vi "Release.vi"(8 "error in (no error)":errorcluster, 11 "Sequence in":refnum<class "Sequence.lvclass">) -> (0 "error out":errorcluster)   [LabVIEW 2020, in "TSnax.lvlib" / "Sequence.lvclass"]
uses:
  Sequence.lvclass
  Sequence.lvclass/Sequence.ctl
  PropertyObject/PropertyObject.lvclass
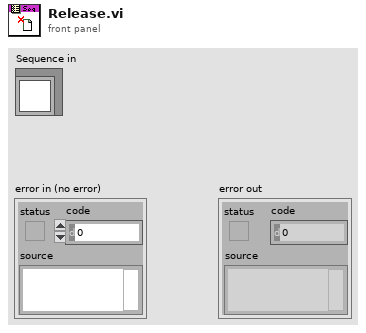
[diagram p1: front panel]
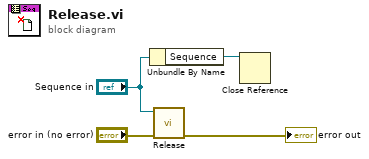
[diagram p0: block diagram]
diagram:
  n1 = Unbundle By Name("Sequence in") -> ("Sequence"=w1:refnum<k7>)
  n2 = call-parent "Release.vi"("error in (no error)"="error in (no error)", "PropertyObject in"="Sequence in") -> ("error out"=→"error out":errorcluster)  [unwired: 9 in]
  n3 = Close Reference(reference=w1) -> ()  [unwired: 1 in, 1 out]
